vi "Trans-RT.vi"() -> ()   [LabVIEW 2016]
uses:
  GP307 cluster.ctl
  <vilib>/Platform/TimedLoop/XDataNode/timing_clust.ctl
  <vilib>/Platform/TimedLoop/XDataNode/nitl_modes.ctl
  <vilib>/Platform/TimedLoop/XDataNode/wakeup.ctl
  <vilib>/FPGAPlugInAG/cRIO-9067/niLvFpga_Open_cRIO-9067.vi
  <vilib>/rvi/errors/niLvFpgaMergeErrorWithErrorCode.vi
  <vilib>/Utility/error.llb/Error Cluster From Error Code.vi
  <vilib>/rvi/errors/niLvFpgaAdjustHostInterfaceError.vi
  <vilib>/functionblocks/Control/PID/PID.vi
  <vilib>/rvi/interface/nirviOpenFPGA/nirviOpenFPGA.xnode
  Slow-Switching-Control/FPGA Bitfiles/Controlsoftware2_FPGATarget4_Trans-FPGA_uDTSqFZP8mU.lvbitx
  Trans-FPGA.vi
  <vilib>/Platform/TimedLoop/XDataNode/XDataNode.xnode
  <vilib>/rvi/interface/nirviReadWriteControl/nirviReadWriteControl.xnode
  <vilib>/functionblocks/FB Core/FB Core.xnode
  <vilib>/functionblocks/FB Property/FB Overlay DBL.ctl
  <vilib>/functionblocks/NI_FunctionBlock Libraries.lvlib
  NiFpgaLv.dll
  <vilib>/Platform/TimedLoop/XDataNode/XDNodeRunTimeDep.lvlib
panel:
  in  "Tab Control":enum32{"Controls/Readbacks", "Errors", "Other"}(tab)
  out "Steerer X+":dbl
  out "Steerer X-":dbl
  out "Steerer Y+":dbl
  out "Steerer Y-":dbl
  out "ExB +":dbl
  out "ExB -":dbl
  out "X+ V":fxp<+/-,26,5> format="%.23g"
  out "X+ I":fxp<+/-,26,5> format="%_4g"
  out "X- V":fxp<+/-,26,5> format="%_4g"
  out "X- I":fxp<+/-,26,5> format="%_4g"
  out "Y+ V":fxp<+/-,26,5> format="%_4g"
  out "Y+ I":fxp<+/-,26,5> format="%_4g"
  out "Y- V":fxp<+/-,26,5> format="%_4g"
  out "Y- I":fxp<+/-,26,5> format="%_4g"
  out "ExB+ V":fxp<+/-,26,5> format="%_4g"
  out "ExB+ I":fxp<+/-,26,5> format="%_4g"
  out "ExB- V":fxp<+/-,26,5> format="%_4g"
  out "ExB- I":fxp<+/-,26,5> format="%_4g"
  out "ExB mag command string":string
  out "Switch object vac gauge cluster":T1
  out "Analyze image vac gauge cluster":T1
  out "EXB":dbl
  in  "derivative time (Td, min) -analyzer":dbl=0.05
  in  "integral time (Ti, min) -analyzer":dbl=0.01
  in  "proportional gain (Kc) -analyzer":dbl=25.0
  out "Analyzer mag command string":string
  out "analyzer field read":dbl
  out "Analyzer mag command":u8[](array[numeric])
  out "Analyzer mag field read":u8[](array[numeric])
  out "Analyzer mag field set":dbl
  in  "output high - analyzer":dbl=300.0
  in  "output low - analyzer":dbl
  out "Switch mag field set":dbl
  out "Switch mag field read":u8[](array[numeric])
  out "switch mag field read":dbl
  out "Switch mag command":u8[](array[numeric])
  in  "derivative time (Td, min) - switch":dbl=0.01
  in  "integral time (Ti, min) - switch":dbl=0.01
  in  "proportional gain (Kc) - switch":dbl=10.0
  out "Switch mag command string":string
  in  "output high - switch":dbl=250.0
  in  "output low - switch":dbl
  out "ExB mag command":u8[](array[numeric])
  out "Ion gauge 1":u8[](array[numeric])
  out "Convectron 1":u8[](array[numeric])
  out "Ion gauge 2":u8[](array[numeric])
  out "Convectron 2":u8[](array[numeric])
  out "Ion gauge 3":u8[](array[numeric])
  out "Convectron 3":u8[](array[numeric])
  out "Ion gauge 4":u8[](array[numeric])
  out "Convectron 4":u8[](array[numeric])
  out "ExB- HV Enable":bool
  out "ExB+ HV Enable":bool
  out "X-steerer+ HV Enable":bool
  out "X-steerer- HV Enable":bool
  out "Y-steerer+ HV Enable":bool
  out "Y-steerer- HV Enable":bool
  out "Readback loop error":errorcluster
  out "Vacuum loop error":errorcluster
  out "Control Loop error":errorcluster
  out "ExB error":errorcluster
  out "Switch Magnet error":errorcluster
  out "Analyzer Magnet error":errorcluster
  in  "Ion gauge cluster control":T2
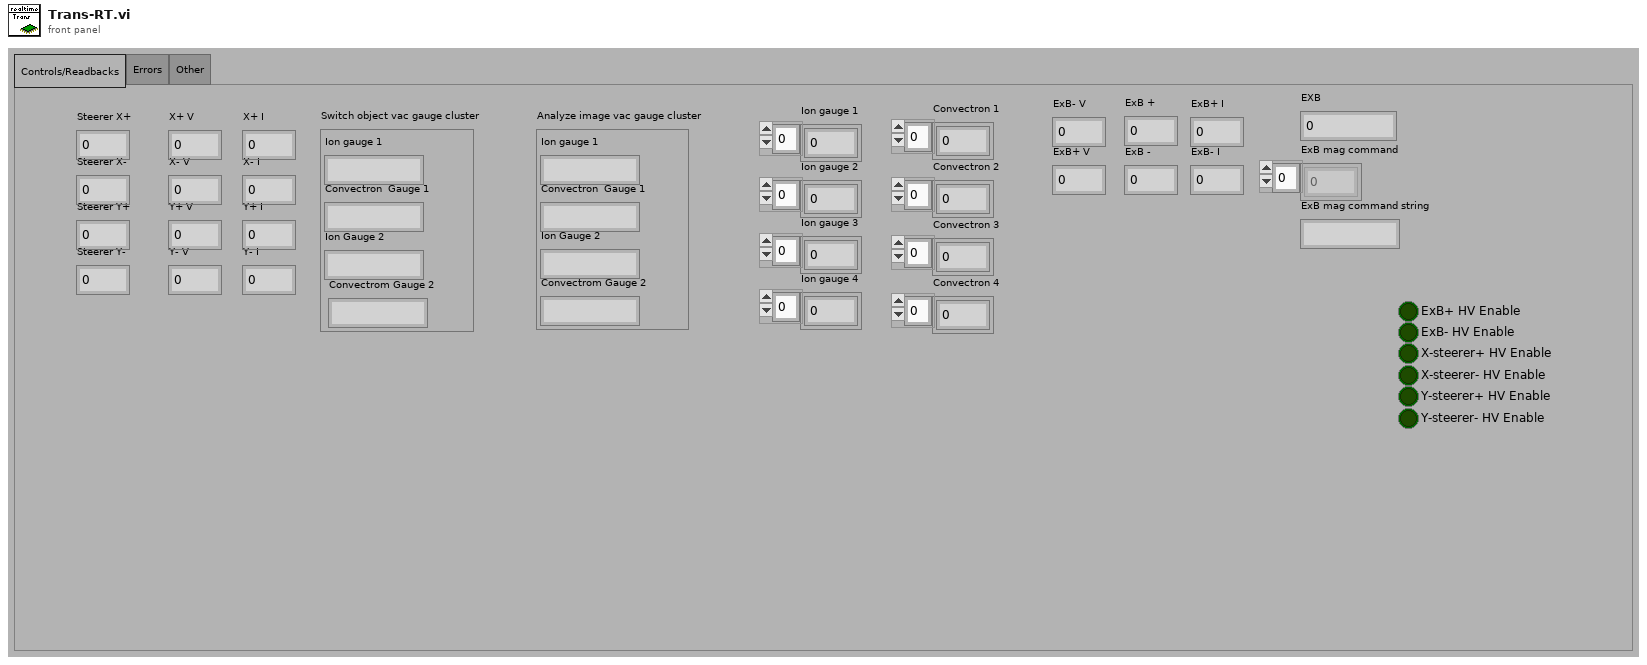
[diagram p1: front panel]
types:
  T1 = cluster{"Ion gauge 1":string, "Convectron  Gauge 1 ":string, "Ion Gauge 2":string, "Convectrom Gauge 2":string}
  T2 = typedef "GP307 cluster.ctl" = cluster{"Ion gauge 1":string, "Convectron  Gauge 1 ":string, "Ion Gauge 2":string, "Convectrom Gauge 2":string}
  T3 = typedef "XDNodeRunTimeDep.lvlib/timing_clust.ctl" = cluster{"Expected End [f-1]":u64, "Actual End [f-1]":u64, "Finished Late? [f-1]":bool, "Expected End [i-1]":u64, "Actual End [i-1]":u64, "Finished Late? [i-1]":bool, "Expected Start [i]":u64, "Actual Start [i]":u64, "Expected Start [f]":u64, "Actual Start [f]":u64, "Source Name":string, "Structure Name":string, "Period":i64, "Deadline":i64, "Offset":i64, "Start":i64, "Priority":i32, "Timeout":i32, "Mode":T4, "Wakeup Reason":T5, "Error":errorcluster, "Source Type":string, "Secondary Source Type":string, "Global End Time":u64, "Global Start Time":u64, "Frame Duration":u64, "Iteration Duration":u64, "Assigned CPU":i32, "I/O Scan Engine Mode":u32}
  T4 = typedef "XDNodeRunTimeDep.lvlib/nitl_modes.ctl" = enum32{"No Change", "Process missed periods, maintain original phase", "Discard missed periods, maintain original phase", "Process missed periods, ignore original phase", "Discard missed periods, ignore original phase"}
  T5 = typedef "XDNodeRunTimeDep.lvlib/wakeup.ctl" = enum32{"Normal", "Aborted", "Asynchronous wakeup", "Timing source error", "Timed loop error", "Timeout"}
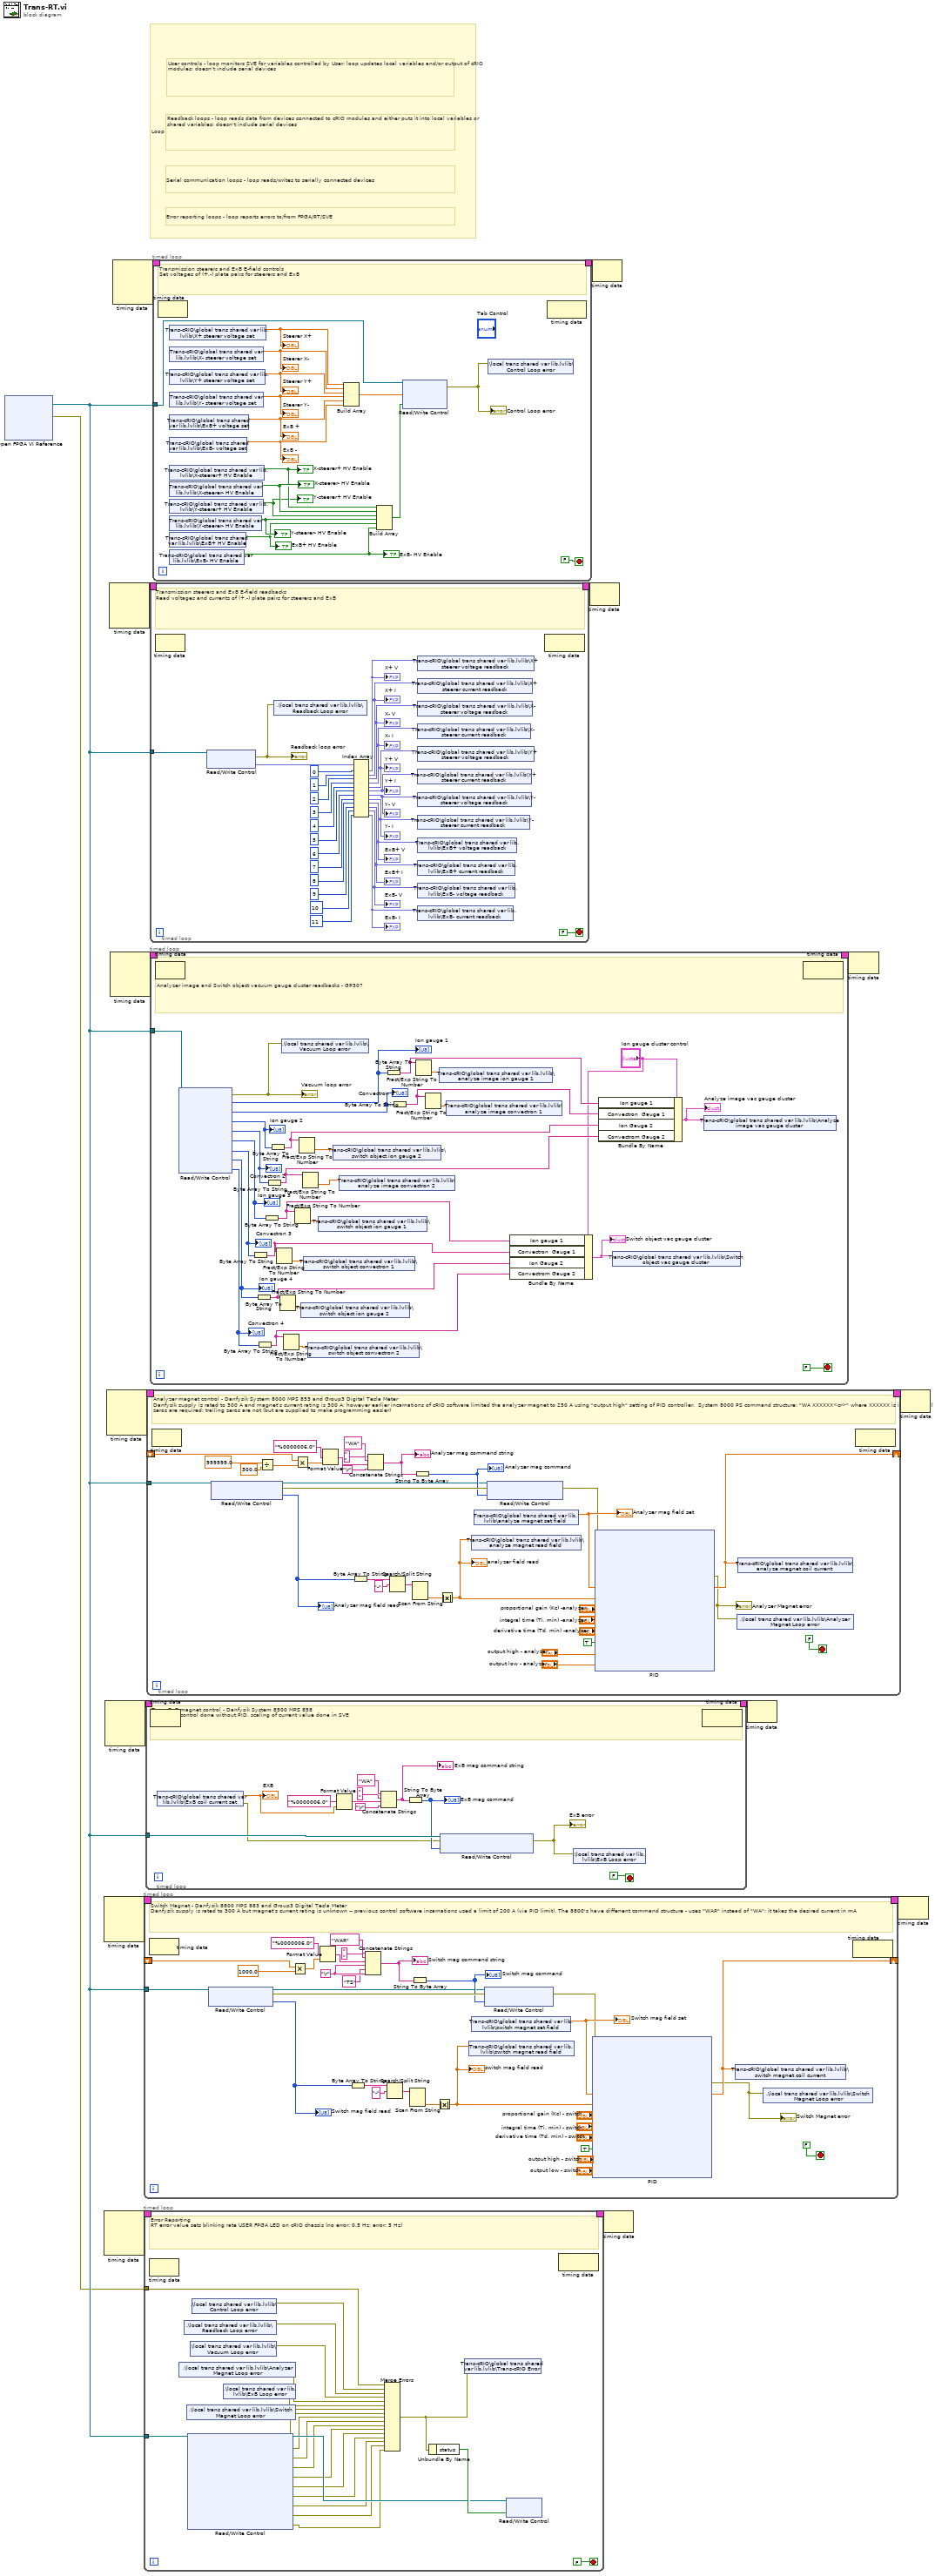
[diagram p0: block diagram]
diagram:
  # "Error reporting loops - loop reports errors to/from FPGA/RT/SVE"
  # "Serial communication loops - loop reads/writes to serially connected devices"
  # "Readback loops - loop reads data from devices connected to cRIO modules and either puts it into local variables or shared variables; doesn't include serial devices"
  # "User controls - loop monitors SVE for variables controlled by User; loop updates local variables and/or output of cRIO modules; doesn't include serial devices"
  # "Loop legend - loops are color coded by responsibility"
  n1 = xnode "Open FPGA VI Reference"() -> ("FPGA VI Reference Out"=w2:refnum<k20>, "error out"=w1:errorcluster)  [unwired: 2 in]
  n2 = node-c288() -> (w6:T3)  [unwired: 4 in]
  n3 = node-c288() -> (w4:T3)  [unwired: 4 in]
  n4 = node-c288() -> (w10:T3)  [unwired: 4 in]
  n5 = node-c288() -> (w12:T3)  [unwired: 4 in]
  n6 = node-c288() -> (w8:T3)  [unwired: 4 in]
  n7 = node-c288() -> (w14:T3)  [unwired: 4 in]
  n8 = node-c288() -> (w16:T3)  [unwired: 4 in]
  n9 = timed-loop {
    shift-right: [w37] -> _
    shift-left: _ -> [w28]
    tunnel: w2 -> [w32]
    timing: w6 -> [_]
    timing-out: [_] -> w5
    stop <- FALSE stop-if-true
    w20 = "\r"
    # "Switch Magnet - Danfysik 8800 MPS 883 and Group3 Digital Tesla Meter\nDanfysik supply is rated to 300 A but magnet's current rating is unknown -- previous control software incarnations used a limit of 200 A (via PID limit). The 8800's have diffenent command structure - uses \"WAR\" instead of \"WA\"; it takes the desired current in mA"
    n10 = node-c288() -> ()  [unwired: 1 in, 1 out]
    n11 = xnode "Read/Write Control"("FPGA VI Reference In"=w32) -> ("FPGA VI Reference Out"=w24:refnum<k20>, "error out"=w31:errorcluster, "switch mag field"=w27:u8[])  [unwired: 1 in]
    "Switch mag field read" <- w27
    n12 = Multiply(x=w28, y=1000.0) -> (x*y=w43:dbl)
    n13 = Format Value(format string="%0000006.0", value (0)=w43) -> (output string=w46:string)  [unwired: 1 out]
    n14 = Byte Array To String(unsigned byte array=w27) -> (string=w39:string)
    n15 = Concatenate Strings("WAR", " ", w46, w20, "TS" ("string"), w20) -> (w47:string)
    "Switch mag command string" <- w47
    n16 = Search/Split String(string=w39, search string/char (-)="-") -> (match + rest of string=w29:string)  [unwired: 3 out]
    n17 = Scan From String(input string=w29) -> (output 1=w38:dbl)  [unwired: 3 in, 4 out]
    n18 = String To Byte Array(string=w47) -> (unsigned byte array=w30:u8[])
    "Switch mag command" <- w30
    n19 = Absolute Value(x=w38) -> (abs(x)=w25:dbl)
    "switch mag field read" <- w25
    n20 = shared-variable "Trans-cRIO\\global trans shared var lib.lvlib\\switch magnet read field"(w25) -> ()  [unwired: 1 in, 1 out]
    n21 = shared-variable "Trans-cRIO\\global trans shared var lib.lvlib\\switch magnet set field"() -> (w26:dbl)  [unwired: 1 in, 1 out]
    "Switch mag field set" <- w26
    n22 = xnode "Read/Write Control"("FPGA VI Reference In"=w24, "error in"=w31, "switch mag ps set"=w30) -> ("error out"=w23:errorcluster)  [unwired: 1 out]
    n23 = xnode "PID"("error in"=w23, "setpoint"=w26, "process variable"=w25, "proportional gain (Kc)"="proportional gain (Kc) - switch", "integral time (Ti, min)"="integral time (Ti, min) - switch", "derivative time (Td, min)"="derivative time (Td, min) - switch", "auto? (T)"=TRUE, "output high"="output high - switch", "output low"="output low - switch") -> ("error out"=w22:errorcluster, "output"=w37:dbl)
    "Switch Magnet error" <- w22
    n24 = shared-variable "Trans-cRIO\\global trans shared var lib.lvlib\\switch magnet coil current"(w37) -> ()  [unwired: 1 in, 1 out]
    n25 = shared-variable ".\\local trans shared var lib.lvlib\\Switch Magnet Loop error"(w22) -> ()  [unwired: 1 in, 1 out]
    n26 = node-c288() -> ()  [unwired: 1 in, 1 out]
  }
  n27 = timed-loop {
    timing: w4 -> [_]
    timing-out: [_] -> w3
    tunnel: w2 -> [w129]
    tunnel: w1 -> [w117]
    stop <- FALSE stop-if-true
    # "Error Reporting\nRT error value sets blinking rate USER FPGA LED on cRIO chassis (no error: 0.5 Hz; error: 5 Hz)"
    n28 = node-c288() -> ()  [unwired: 1 in, 1 out]
    n29 = shared-variable ".\\local trans shared var lib.lvlib\\Analyzer Magnet Loop error"() -> (w132:errorcluster)  [unwired: 1 in, 1 out]
    n30 = shared-variable ".\\local trans shared var lib.lvlib\\Readback Loop error"() -> (w134:errorcluster)  [unwired: 1 in, 1 out]
    n31 = shared-variable ".\\local trans shared var lib.lvlib\\Switch Magnet Loop error"() -> (w130:errorcluster)  [unwired: 1 in, 1 out]
    n32 = xnode "Read/Write Control"("FPGA VI Reference In"=w129) -> ("FPGA VI Reference Out"=w128:refnum<k20>, "error out"=w127:errorcluster, "9205 error"=w126:errorcluster, "9264 error"=w125:errorcluster, "Analyzer PS error"=w124:errorcluster, "ExB PS error"=w123:errorcluster, "Switch PS error"=w122:errorcluster, "Analyzer Hall Probe error"=w121:errorcluster, "Switch Hall Probe error"=w120:errorcluster, "Analyze Image Vacuum Error"=w119:errorcluster, "Switch Object Vacuum Error"=w118:errorcluster)  [unwired: 1 in]
    n33 = shared-variable ".\\local trans shared var lib.lvlib\\Vacuum Loop error"() -> (w133:errorcluster)  [unwired: 1 in, 1 out]
    n34 = shared-variable ".\\local trans shared var lib.lvlib\\Control Loop error"() -> (w135:errorcluster)  [unwired: 1 in, 1 out]
    n35 = shared-variable ".\\local trans shared var lib.lvlib\\ExB Loop error"() -> (w131:errorcluster)  [unwired: 1 in, 1 out]
    n36 = Merge Errors(w117, w135, w134, w133, w132, w131, w130, w127, w126, w125, w124, w123, w122, w121, w120, w119, w118) -> (w137:errorcluster)
    n37 = Unbundle By Name(w137) -> ("status"=w136:bool)
    n38 = shared-variable "Trans-cRIO\\global trans shared var lib.lvlib\\Trans-cRIO Error"(w137) -> ()  [unwired: 1 in, 1 out]
    n39 = xnode "Read/Write Control"("FPGA VI Reference In"=w128, "RT error"=w136) -> ()  [unwired: 1 in, 2 out]
    n40 = node-c288() -> ()  [unwired: 1 in, 1 out]
  }
  n41 = timed-loop {
    timing: w10 -> [_]
    timing-out: [_] -> w9
    tunnel: w2 -> [w144]
    stop <- FALSE stop-if-true
    # "Trans ExB magnet control - Danfysik System 8500 MPS 858\nSince ExB control done without PID, scaling of current value done in SVE"
    n42 = node-c288() -> ()  [unwired: 1 in, 1 out]
    n43 = shared-variable "Trans-cRIO\\global trans shared var lib.lvlib\\ExB coil current set"() -> (w141:dbl, error out=w140:errorcluster)  [unwired: 1 in]
    "EXB" <- w141
    n44 = Format Value(format string="%0000006.0", value (0)=w141) -> (output string=w148:string)  [unwired: 1 out]
    n45 = Concatenate Strings("WA", " ", w148, "\r") -> (w145:string)
    "ExB mag command string" <- w145
    n46 = String To Byte Array(string=w145) -> (unsigned byte array=w142:u8[])
    "ExB mag command" <- w142
    n47 = xnode "Read/Write Control"("FPGA VI Reference In"=w144, "error in"=w140, "trans ExB mag ps set"=w142) -> ("error out"=w143:errorcluster)  [unwired: 1 out]
    "ExB error" <- w143
    n48 = shared-variable ".\\local trans shared var lib.lvlib\\ExB Loop error"(w143) -> ()  [unwired: 1 in, 1 out]
    n49 = node-c288() -> ()  [unwired: 1 in, 1 out]
  }
  n50 = timed-loop {
    shift-right: [w171] -> _
    shift-left: _ -> [w162]
    tunnel: w2 -> [w166]
    timing: w12 -> [_]
    timing-out: [_] -> w11
    stop <- FALSE stop-if-true
    # "Analyzer magnet control - Danfysik System 8000 MPS 853 and Group3 Digital Tesla Meter\nDanfysik supply is rated to 300 A and magnet's current rating is 300 A; however earlier incarnations of cRIO software limited the analyzer magnet to 250 A using \"output high\" setting of PID controller.  System 8000 PS command structure: \"WA XXXXXX<cr>\" where XXXXXX is in PPM of full current. Leading zeros are required; trailing zeros are not (but are supplied to make programming easier)"
    n51 = node-c288() -> ()  [unwired: 1 in, 1 out]
    n52 = xnode "Read/Write Control"("FPGA VI Reference In"=w166) -> ("FPGA VI Reference Out"=w158:refnum<k20>, "error out"=w165:errorcluster, "analyzer mag field"=w161:u8[])  [unwired: 1 in]
    "Analyzer mag field read" <- w161
    n53 = Divide(x=999999.0, y=300.0) -> (x/y=w178:dbl)
    n54 = Multiply(x=w162, y=w178) -> (x*y=w180:dbl)
    n55 = Format Value(format string="%0000006.0", value (0)=w180) -> (output string=w183:string)  [unwired: 1 out]
    n56 = Byte Array To String(unsigned byte array=w161) -> (string=w173:string)
    n57 = Concatenate Strings("WA", " ", w183, "\r") -> (w184:string)
    "Analyzer mag command string" <- w184
    n58 = Search/Split String(string=w173, search string/char (-)="-") -> (match + rest of string=w163:string)  [unwired: 3 out]
    n59 = Scan From String(input string=w163) -> (output 1=w172:dbl)  [unwired: 3 in, 4 out]
    n60 = String To Byte Array(string=w184) -> (unsigned byte array=w164:u8[])
    "Analyzer mag command" <- w164
    n61 = Absolute Value(x=w172) -> (abs(x)=w159:dbl)
    "analyzer field read" <- w159
    n62 = shared-variable "Trans-cRIO\\global trans shared var lib.lvlib\\analyze magnet read field"(w159) -> ()  [unwired: 1 in, 1 out]
    n63 = shared-variable "Trans-cRIO\\global trans shared var lib.lvlib\\analyze magnet set field"() -> (w160:dbl)  [unwired: 1 in, 1 out]
    "Analyzer mag field set" <- w160
    n64 = xnode "Read/Write Control"("FPGA VI Reference In"=w158, "error in"=w165, "analyzer mag ps set"=w164) -> ("error out"=w157:errorcluster)  [unwired: 1 out]
    n65 = xnode "PID"("error in"=w157, "setpoint"=w160, "process variable"=w159, "proportional gain (Kc)"="proportional gain (Kc) -analyzer", "integral time (Ti, min)"="integral time (Ti, min) -analyzer", "derivative time (Td, min)"="derivative time (Td, min) -analyzer", "auto? (T)"=TRUE, "output high"="output high - analyzer", "output low"="output low - analyzer") -> ("error out"=w156:errorcluster, "output"=w171:dbl)
    "Analyzer Magnet error" <- w156
    n66 = shared-variable ".\\local trans shared var lib.lvlib\\Analyzer Magnet Loop error"(w156) -> ()  [unwired: 1 in, 1 out]
    n67 = shared-variable "Trans-cRIO\\global trans shared var lib.lvlib\\analyze magnet coil current"(w171) -> ()  [unwired: 1 in, 1 out]
    n68 = node-c288() -> ()  [unwired: 1 in, 1 out]
  }
  n69 = timed-loop {
    timing: w8 -> [_]
    timing-out: [_] -> w7
    tunnel: w2 -> [w255]
    stop <- FALSE stop-if-true
    # "Transmission steerers and ExB E-field readbacks\nRead voltages and currents of (+,-) plate pairs for steerers and ExB"
    n70 = node-c288() -> ()  [unwired: 1 in, 1 out]
    n71 = xnode "Read/Write Control"("FPGA VI Reference In"=w255) -> ("error out"=w254:errorcluster, "HV monitor"=w281:fxp<+/-,26,5>[])  [unwired: 1 in, 1 out]
    "Readback loop error" <- w254
    n72 = shared-variable ".\\local trans shared var lib.lvlib\\Readback Loop error"(w254) -> ()  [unwired: 1 in, 1 out]
    n73 = Index Array(array=w281, index #1=0 ("index"), index #2=1 ("index"), index #3=2 ("index"), index #4=3 ("index"), index #5=4 ("index"), index #6=5 ("index"), index #7=6 ("index"), index #8=7 ("index"), index #9=8 ("index"), index #10=9 ("index"), index #11=10 ("index"), index #12=11 ("index")) -> (element #1=w270:fxp<+/-,26,5>, element #2=w272:fxp<+/-,26,5>, element #3=w271:fxp<+/-,26,5>, element #4=w269:fxp<+/-,26,5>, element #5=w273:fxp<+/-,26,5>, element #6=w275:fxp<+/-,26,5>, element #7=w274:fxp<+/-,26,5>, element #8=w276:fxp<+/-,26,5>, element #9=w277:fxp<+/-,26,5>, element #10=w279:fxp<+/-,26,5>, element #11=w278:fxp<+/-,26,5>, element #12=w280:fxp<+/-,26,5>)
    "X+ V" <- w270
    "X+ I" <- w272
    "X- V" <- w271
    "X- I" <- w269
    "Y+ V" <- w273
    "Y+ I" <- w275
    "Y- V" <- w274
    "Y- I" <- w276
    "ExB+ V" <- w277
    "ExB+ I" <- w279
    "ExB- V" <- w278
    "ExB- I" <- w280
    n74 = shared-variable "Trans-cRIO\\global trans shared var lib.lvlib\\X+ steerer voltage readback"(w270) -> ()  [unwired: 1 in, 1 out]
    n75 = shared-variable "Trans-cRIO\\global trans shared var lib.lvlib\\X+ steerer current readback"(w272) -> ()  [unwired: 1 in, 1 out]
    n76 = shared-variable "Trans-cRIO\\global trans shared var lib.lvlib\\X- steerer voltage readback"(w271) -> ()  [unwired: 1 in, 1 out]
    n77 = shared-variable "Trans-cRIO\\global trans shared var lib.lvlib\\X- steerer current readback"(w269) -> ()  [unwired: 1 in, 1 out]
    n78 = shared-variable "Trans-cRIO\\global trans shared var lib.lvlib\\Y+ steerer voltage readback"(w273) -> ()  [unwired: 1 in, 1 out]
    n79 = shared-variable "Trans-cRIO\\global trans shared var lib.lvlib\\Y+ steerer current readback"(w275) -> ()  [unwired: 1 in, 1 out]
    n80 = shared-variable "Trans-cRIO\\global trans shared var lib.lvlib\\Y- steerer voltage readback"(w274) -> ()  [unwired: 1 in, 1 out]
    n81 = shared-variable "Trans-cRIO\\global trans shared var lib.lvlib\\Y- steerer current readback"(w276) -> ()  [unwired: 1 in, 1 out]
    n82 = shared-variable "Trans-cRIO\\global trans shared var lib.lvlib\\ExB+ voltage readback"(w277) -> ()  [unwired: 1 in, 1 out]
    n83 = shared-variable "Trans-cRIO\\global trans shared var lib.lvlib\\ExB+ current readback"(w279) -> ()  [unwired: 1 in, 1 out]
    n84 = shared-variable "Trans-cRIO\\global trans shared var lib.lvlib\\ExB- voltage readback"(w278) -> ()  [unwired: 1 in, 1 out]
    n85 = shared-variable "Trans-cRIO\\global trans shared var lib.lvlib\\ExB- current readback"(w280) -> ()  [unwired: 1 in, 1 out]
    n86 = node-c288() -> ()  [unwired: 1 in, 1 out]
  }
  n87 = timed-loop {
    tunnel: w2 -> [w289]
    timing: w14 -> [_]
    timing-out: [_] -> w13
    stop <- FALSE stop-if-true
    # "Analyzer image and Switch object vacuum gauge cluster readbacks - GP307"
    n88 = node-c288() -> ()  [unwired: 1 in, 1 out]
    n89 = xnode "Read/Write Control"("FPGA VI Reference In"=w289) -> ("error out"=w288:errorcluster, "Ion gauge 1"=w310:u8[], "Convectron 1"=w311:u8[], "Ion gauge 2"=w312:u8[], "Convectron 2"=w313:u8[], "Ion gauge 3"=w308:u8[], "Convectron 3"=w307:u8[], "Ion gauge 4"=w286:u8[], "Convectron 4"=w285:u8[])  [unwired: 1 in, 1 out]
    "Vacuum loop error" <- w288
    "Ion gauge 1" <- w310
    "Convectron 1" <- w311
    "Ion gauge 2" <- w312
    "Convectron 2" <- w313
    "Ion gauge 3" <- w308
    "Convectron 3" <- w307
    "Ion gauge 4" <- w286
    "Convectron 4" <- w285
    n90 = Byte Array To String(unsigned byte array=w307) -> (string=w304:string)
    n91 = Byte Array To String(unsigned byte array=w286) -> (string=w303:string)
    n92 = Byte Array To String(unsigned byte array=w285) -> (string=w302:string)
    n93 = Byte Array To String(unsigned byte array=w308) -> (string=w305:string)
    n94 = Byte Array To String(unsigned byte array=w313) -> (string=w295:string)
    n95 = Byte Array To String(unsigned byte array=w312) -> (string=w294:string)
    n96 = Fract/Exp String To Number(string=w304) -> (number=w300:dbl)  [unwired: 3 in, 1 out]
    n97 = Fract/Exp String To Number(string=w303) -> (number=w299:dbl)  [unwired: 3 in, 1 out]
    n98 = shared-variable ".\\local trans shared var lib.lvlib\\Vacuum Loop error"(w288) -> ()  [unwired: 1 in, 1 out]
    n99 = Fract/Exp String To Number(string=w302) -> (number=w298:dbl)  [unwired: 3 in, 1 out]
    n100 = Fract/Exp String To Number(string=w305) -> (number=w301:dbl)  [unwired: 3 in, 1 out]
    n101 = Fract/Exp String To Number(string=w294) -> (number=w292:dbl)  [unwired: 3 in, 1 out]
    n102 = shared-variable "Trans-cRIO\\global trans shared var lib.lvlib\\switch object ion gauge 2"(w299) -> ()  [unwired: 1 in, 1 out]
    n103 = Fract/Exp String To Number(string=w295) -> (number=w290:dbl)  [unwired: 3 in, 1 out]
    n104 = shared-variable "Trans-cRIO\\global trans shared var lib.lvlib\\switch object convectron 1"(w300) -> ()  [unwired: 1 in, 1 out]
    n105 = shared-variable "Trans-cRIO\\global trans shared var lib.lvlib\\switch object convectron 2"(w298) -> ()  [unwired: 1 in, 1 out]
    n106 = shared-variable "Trans-cRIO\\global trans shared var lib.lvlib\\switch object ion gauge 1"(w301) -> ()  [unwired: 1 in, 1 out]
    n107 = shared-variable "Trans-cRIO\\global trans shared var lib.lvlib\\switch object ion gauge 2"(w292) -> ()  [unwired: 1 in, 1 out]
    n108 = shared-variable "Trans-cRIO\\global trans shared var lib.lvlib\\analyze image convectron 2"(w290) -> ()  [unwired: 1 in, 1 out]
    n109 = Byte Array To String(unsigned byte array=w310) -> (string=w297:string)
    n110 = Byte Array To String(unsigned byte array=w311) -> (string=w296:string)
    n111 = Fract/Exp String To Number(string=w297) -> (number=w293:dbl)  [unwired: 3 in, 1 out]
    n112 = Fract/Exp String To Number(string=w296) -> (number=w291:dbl)  [unwired: 3 in, 1 out]
    n113 = shared-variable "Trans-cRIO\\global trans shared var lib.lvlib\\analyze image ion gauge 1"(w293) -> ()  [unwired: 1 in, 1 out]
    n114 = shared-variable "Trans-cRIO\\global trans shared var lib.lvlib\\analyze image convectron 1"(w291) -> ()  [unwired: 1 in, 1 out]
    n115 = Bundle By Name(cluster="Ion gauge cluster control", "Ion gauge 1"=w305, "Convectron  Gauge 1"=w304, "Ion Gauge 2"=w303, "Convectrom Gauge 2"=w302) -> (w306:T2)
    "Switch object vac gauge cluster" <- w306
    n116 = Bundle By Name(cluster="Ion gauge cluster control", "Ion gauge 1"=w297, "Convectron  Gauge 1"=w296, "Ion Gauge 2"=w294, "Convectrom Gauge 2"=w295) -> (w287:T2)
    "Analyze image vac gauge cluster" <- w287
    n117 = shared-variable "Trans-cRIO\\global trans shared var lib.lvlib\\Switch object vac gauge cluster"(w306) -> ()  [unwired: 1 in, 1 out]
    n118 = shared-variable "Trans-cRIO\\global trans shared var lib.lvlib\\Analyze image vac gauge cluster"(w287) -> ()  [unwired: 1 in, 1 out]
    n119 = node-c288() -> ()  [unwired: 1 in, 1 out]
  }
  n120 = timed-loop {
    tunnel: w2 -> [w323]
    timing: w16 -> [_]
    timing-out: [_] -> w15
    stop <- FALSE stop-if-true
    # "Transmission steerers and ExB E-field controls\nSet voltages of (+,-) plate pairs for steerers and ExB"
    n121 = node-c288() -> ()  [unwired: 1 in, 1 out]
    n122 = shared-variable "Trans-cRIO\\global trans shared var lib.lvlib\\X-steerer+ HV Enable"() -> (w318:bool)  [unwired: 1 in, 1 out]
    "X-steerer+ HV Enable" <- w318
    n123 = shared-variable "Trans-cRIO\\global trans shared var lib.lvlib\\X-steerer- HV Enable"() -> (w319:bool)  [unwired: 1 in, 1 out]
    "X-steerer- HV Enable" <- w319
    n124 = shared-variable "Trans-cRIO\\global trans shared var lib.lvlib\\Y-steerer+ HV Enable"() -> (w316:bool)  [unwired: 1 in, 1 out]
    "Y-steerer+ HV Enable" <- w316
    n125 = shared-variable "Trans-cRIO\\global trans shared var lib.lvlib\\Y-steerer- HV Enable"() -> (w320:bool)  [unwired: 1 in, 1 out]
    "Y-steerer- HV Enable" <- w320
    n126 = shared-variable "Trans-cRIO\\global trans shared var lib.lvlib\\ExB+ HV Enable"() -> (w317:bool)  [unwired: 1 in, 1 out]
    "ExB+ HV Enable" <- w317
    n127 = shared-variable "Trans-cRIO\\global trans shared var lib.lvlib\\ExB- HV Enable"() -> (w321:bool)  [unwired: 1 in, 1 out]
    "ExB- HV Enable" <- w321
    n128 = shared-variable "Trans-cRIO\\global trans shared var lib.lvlib\\X+ steerer voltage set"() -> (w325:dbl)  [unwired: 1 in, 1 out]
    "Steerer X+" <- w325
    n129 = shared-variable "Trans-cRIO\\global trans shared var lib.lvlib\\X- steerer voltage set"() -> (w326:dbl)  [unwired: 1 in, 1 out]
    "Steerer X-" <- w326
    n130 = shared-variable "Trans-cRIO\\global trans shared var lib.lvlib\\Y+ steerer voltage set"() -> (w327:dbl)  [unwired: 1 in, 1 out]
    "Steerer Y+" <- w327
    n131 = shared-variable "Trans-cRIO\\global trans shared var lib.lvlib\\Y- steerer voltage set"() -> (w328:dbl)  [unwired: 1 in, 1 out]
    "Steerer Y-" <- w328
    n132 = shared-variable "Trans-cRIO\\global trans shared var lib.lvlib\\ExB+ voltage set"() -> (w329:dbl)  [unwired: 1 in, 1 out]
    "ExB +" <- w329
    n133 = shared-variable "Trans-cRIO\\global trans shared var lib.lvlib\\ExB- voltage set"() -> (w330:dbl)  [unwired: 1 in, 1 out]
    "ExB -" <- w330
    n134 = Build Array(w325, w326, w327, w328, w329, w330) -> (w332:dbl[])
    n135 = Build Array(w318, w319, w316, w320, w317, w321) -> (w322:bool[])
    n136 = xnode "Read/Write Control"("FPGA VI Reference In"=w323, "HV Set"=w332, "HV Enable"=w322) -> ("error out"=w324:errorcluster)  [unwired: 1 in, 1 out]
    "Control Loop error" <- w324
    n137 = shared-variable ".\\local trans shared var lib.lvlib\\Control Loop error"(w324) -> ()  [unwired: 1 in, 1 out]
    n138 = node-c288() -> ()  [unwired: 1 in, 1 out]
  }
  n139 = node-c288(w7) -> ()  [unwired: 1 out]
  n140 = node-c288(w15) -> ()  [unwired: 1 out]
  n141 = node-c288(w3) -> ()  [unwired: 1 out]
  n142 = node-c288(w9) -> ()  [unwired: 1 out]
  n143 = node-c288(w13) -> ()  [unwired: 1 out]
  n144 = node-c288(w5) -> ()  [unwired: 1 out]
  n145 = node-c288(w11) -> ()  [unwired: 1 out]
